vi "PythonConverter_BD.vi"(5 "Build Directory":path, 6 "error in":errorcluster, 9 "VI Interpreter in":refnum<class "VI Interpreter.lvclass">) -> (0 "error out":errorcluster, 3 "PythonConverter_BD out":refnum<class "PyConvBD.lvclass">)   [LabVIEW 2014, in "PyConvBD.lvclass"]
uses:
  PyConvBD.lvclass
  VI Interpreter/Classes/VI Interpreter/VI Interpreter.lvclass
  PyConvBD.lvclass/PyConvBD.ctl
  Parsing/Python Functions.lvlib
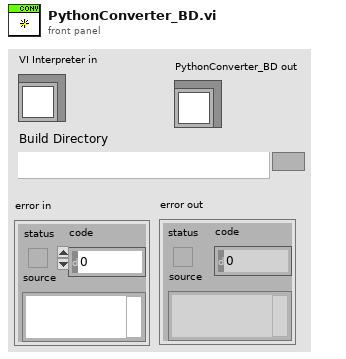
[diagram p1: front panel]
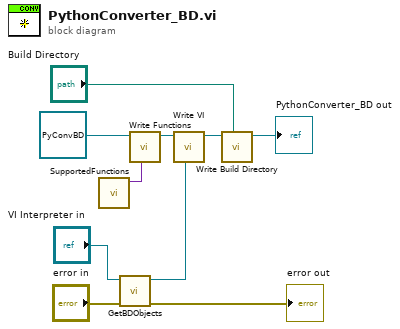
[diagram p0: block diagram]
diagram:
  n1 = call "SupportedFunctions.vi"() -> ("supported functions"=w1:variant)  [unwired: 11 in]
  n2 = call "GetBDObjects.vi"("error in"="error in", "VI Interpreter in"="VI Interpreter in") -> ("error out"=→"error out":errorcluster, "VI Interpreter out"=w7:refnum<class "VI Interpreter.lvclass">)  [unwired: 8 in]
  n3 = call "Write Functions.vi"("Functions"=w1, "PythonConverter_BD in"=refnum<class "PyConvBD.lvclass"> refnum ("PythonConverter_BD out")) -> ("PythonConverter_BD out"=w2:refnum<class "PyConvBD.lvclass">)  [unwired: 7 in]
  n4 = call "Write VI.vi"("VI Interpreter"=w7, "PythonConverter_BD in"=w2) -> ("PythonConverter_BD out"=w6:refnum<class "PyConvBD.lvclass">)  [unwired: 7 in]
  n5 = call "Write Build Directory.vi"("Build Directory"="Build Directory", "PythonConverter_BD in"=w6) -> ("PythonConverter_BD out"=→"PythonConverter_BD out":refnum<class "PyConvBD.lvclass">)  [unwired: 7 in]
